vi "ulysses16.vi"() -> ()   [LabVIEW 2015]
uses:
  TSP Library/TypeDef/Coordinate.ctl
  TSP Library/TSP Library.lvlib
panel:
  out "Distance Select":dbl
  out "Distance My":dbl
  in  "Tour My":u16[](array[numeric])=[1, 16, 12, 13, 14, 6, 7, 10, 9, 11, 5, 15, 8, 4, 2, 3, 1]
  in  "Tour Select":u16[](array[numeric])=[1, 14, 13, 12, 7, 6, 15, 5, 11, 9, 10, 16, 3, 2, 4, 8, 1]
  in  "Coordinate Load":T1[](array[typedef])=[{"x"=38.24, "y"=20.42}, {"x"=39.57, "y"=26.15}, {"x"=40.56, "y"=25.32}, {"x"=36.26, "y"=23.12}, {"x"=33.48, "y"=10.54}, {"x"=37.56, "y"=12.19}, {"x"=38.42, "y"=13.11}, {"x"=37.52, "y"=20.44}, {"x"=41.23, "y"=9.1}, {"x"=41.17, "y"=13.05}, {"x"=36.08, "y"=-5.21}, {"x"=38.47, "y"=15.13}, {"x"=38.15, "y"=15.35}, {"x"=37.51, "y"=15.17}, {"x"=35.49, "y"=14.32}, {"x"=39.36, "y"=19.56}]
  out "Tour's":cluster{dbl[], dbl[]}[](graph)
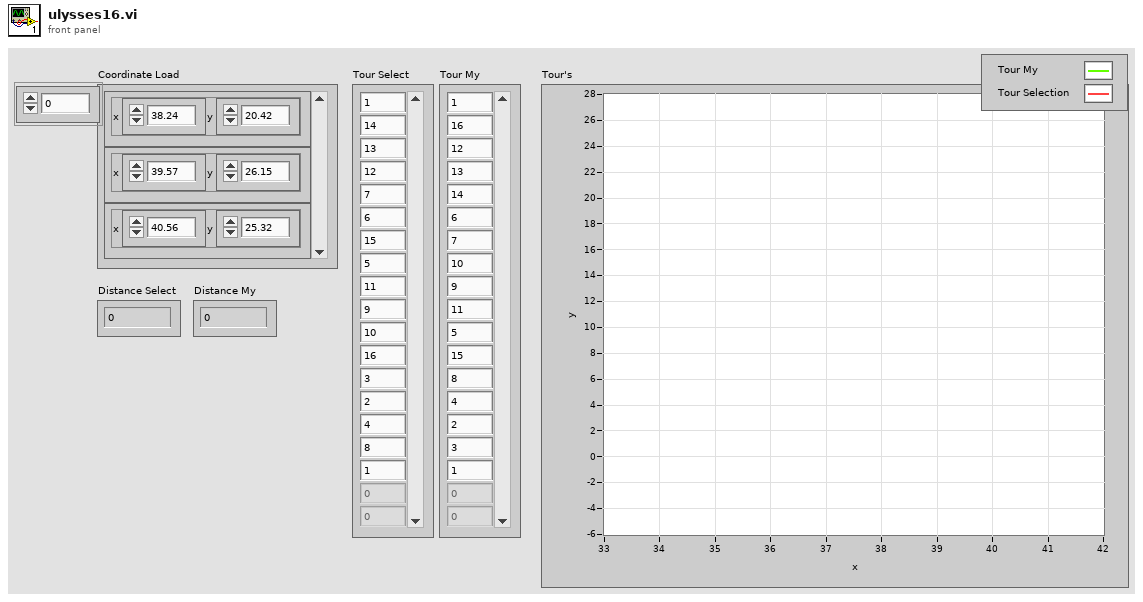
[diagram p1: front panel]
types:
  T1 = typedef "TSP Library.lvlib/Coordinate.ctl" = cluster{"x":dbl, "y":dbl}
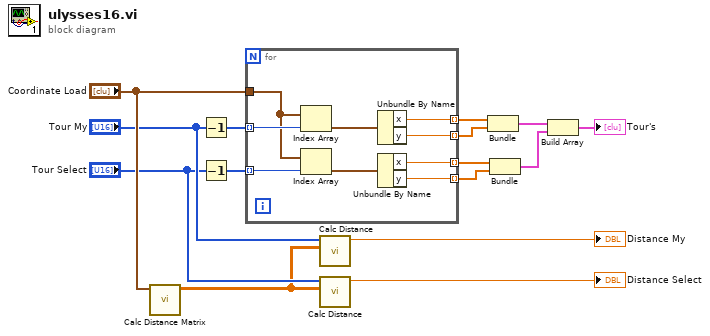
[diagram p0: block diagram]
diagram:
  n1 = call "Calc Distance Matrix.vi"("Coordinate[]"="Coordinate Load") -> ("Distance Matrix"=w2:dbl[][])  [unwired: 10 in]
  n2 = Decrement(x="Tour My") -> (x-1=w15:u16[])
  n3 = Decrement(x="Tour Select") -> (x-1=w14:u16[])
  n4 = for {
    tunnel: "Coordinate Load" -> [w20]
    tunnel: w14 -> [w24] mode=indexing
    tunnel: w15 -> [w23] mode=indexing
    tunnel: [w19] -> w13 mode=indexing
    tunnel: [w18] -> w12 mode=indexing
    tunnel: [w17] -> w9 mode=indexing
    tunnel: [w16] -> w7 mode=indexing
    n5 = Index Array(array=w20, index=w23) -> (element=w22:T1)
    n6 = Index Array(array=w20, index=w24) -> (element=w21:T1)
    n7 = Unbundle By Name(w22) -> ("x"=w19:dbl, "y"=w17:dbl)
    n8 = Unbundle By Name(w21) -> ("x"=w18:dbl, "y"=w16:dbl)
  }
  n9 = call "Calc Distance.vi"("Distance Matrix"=w2, "Tour"="Tour My") -> ("Distance"=→"Distance My":dbl)  [unwired: 9 in]
  n10 = call "Calc Distance.vi"("Distance Matrix"=w2, "Tour"="Tour Select") -> ("Distance"=→"Distance Select":dbl)  [unwired: 9 in]
  n11 = Bundle(w13, w9) -> (w10:cluster{dbl[], dbl[]})  [unwired: 1 in]
  n12 = Bundle(w12, w7) -> (w8:cluster{dbl[], dbl[]})  [unwired: 1 in]
  n13 = Build Array(w10, w8) -> (→"Tour's":cluster{dbl[], dbl[]}[])
